vi "OP600ZP_GlobalVariables.vi"() -> ()   [LabVIEW 2020]
uses:
  CheminDeBase.vi
  <vilib>/Utility/config.llb/Read Key (Double).vi
  OP600ZP_VGConf.vi
  <vilib>/Utility/config.llb/Read Key (String).vi
  OP500/SubVI/OP500ZP_VGConf.vi
  <vilib>/Utility/config.llb/NI_LVConfig.lvlib
panel:
  out "error out 2":errorcluster caption="error out"
  out "error out":errorcluster
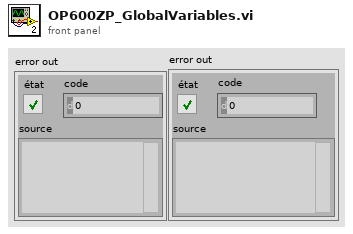
[diagram p1: front panel]
types:
  T1 = typedef "NI_LVConfig.lvlib/Config Data RefNum.ctl" = refnum<k1>
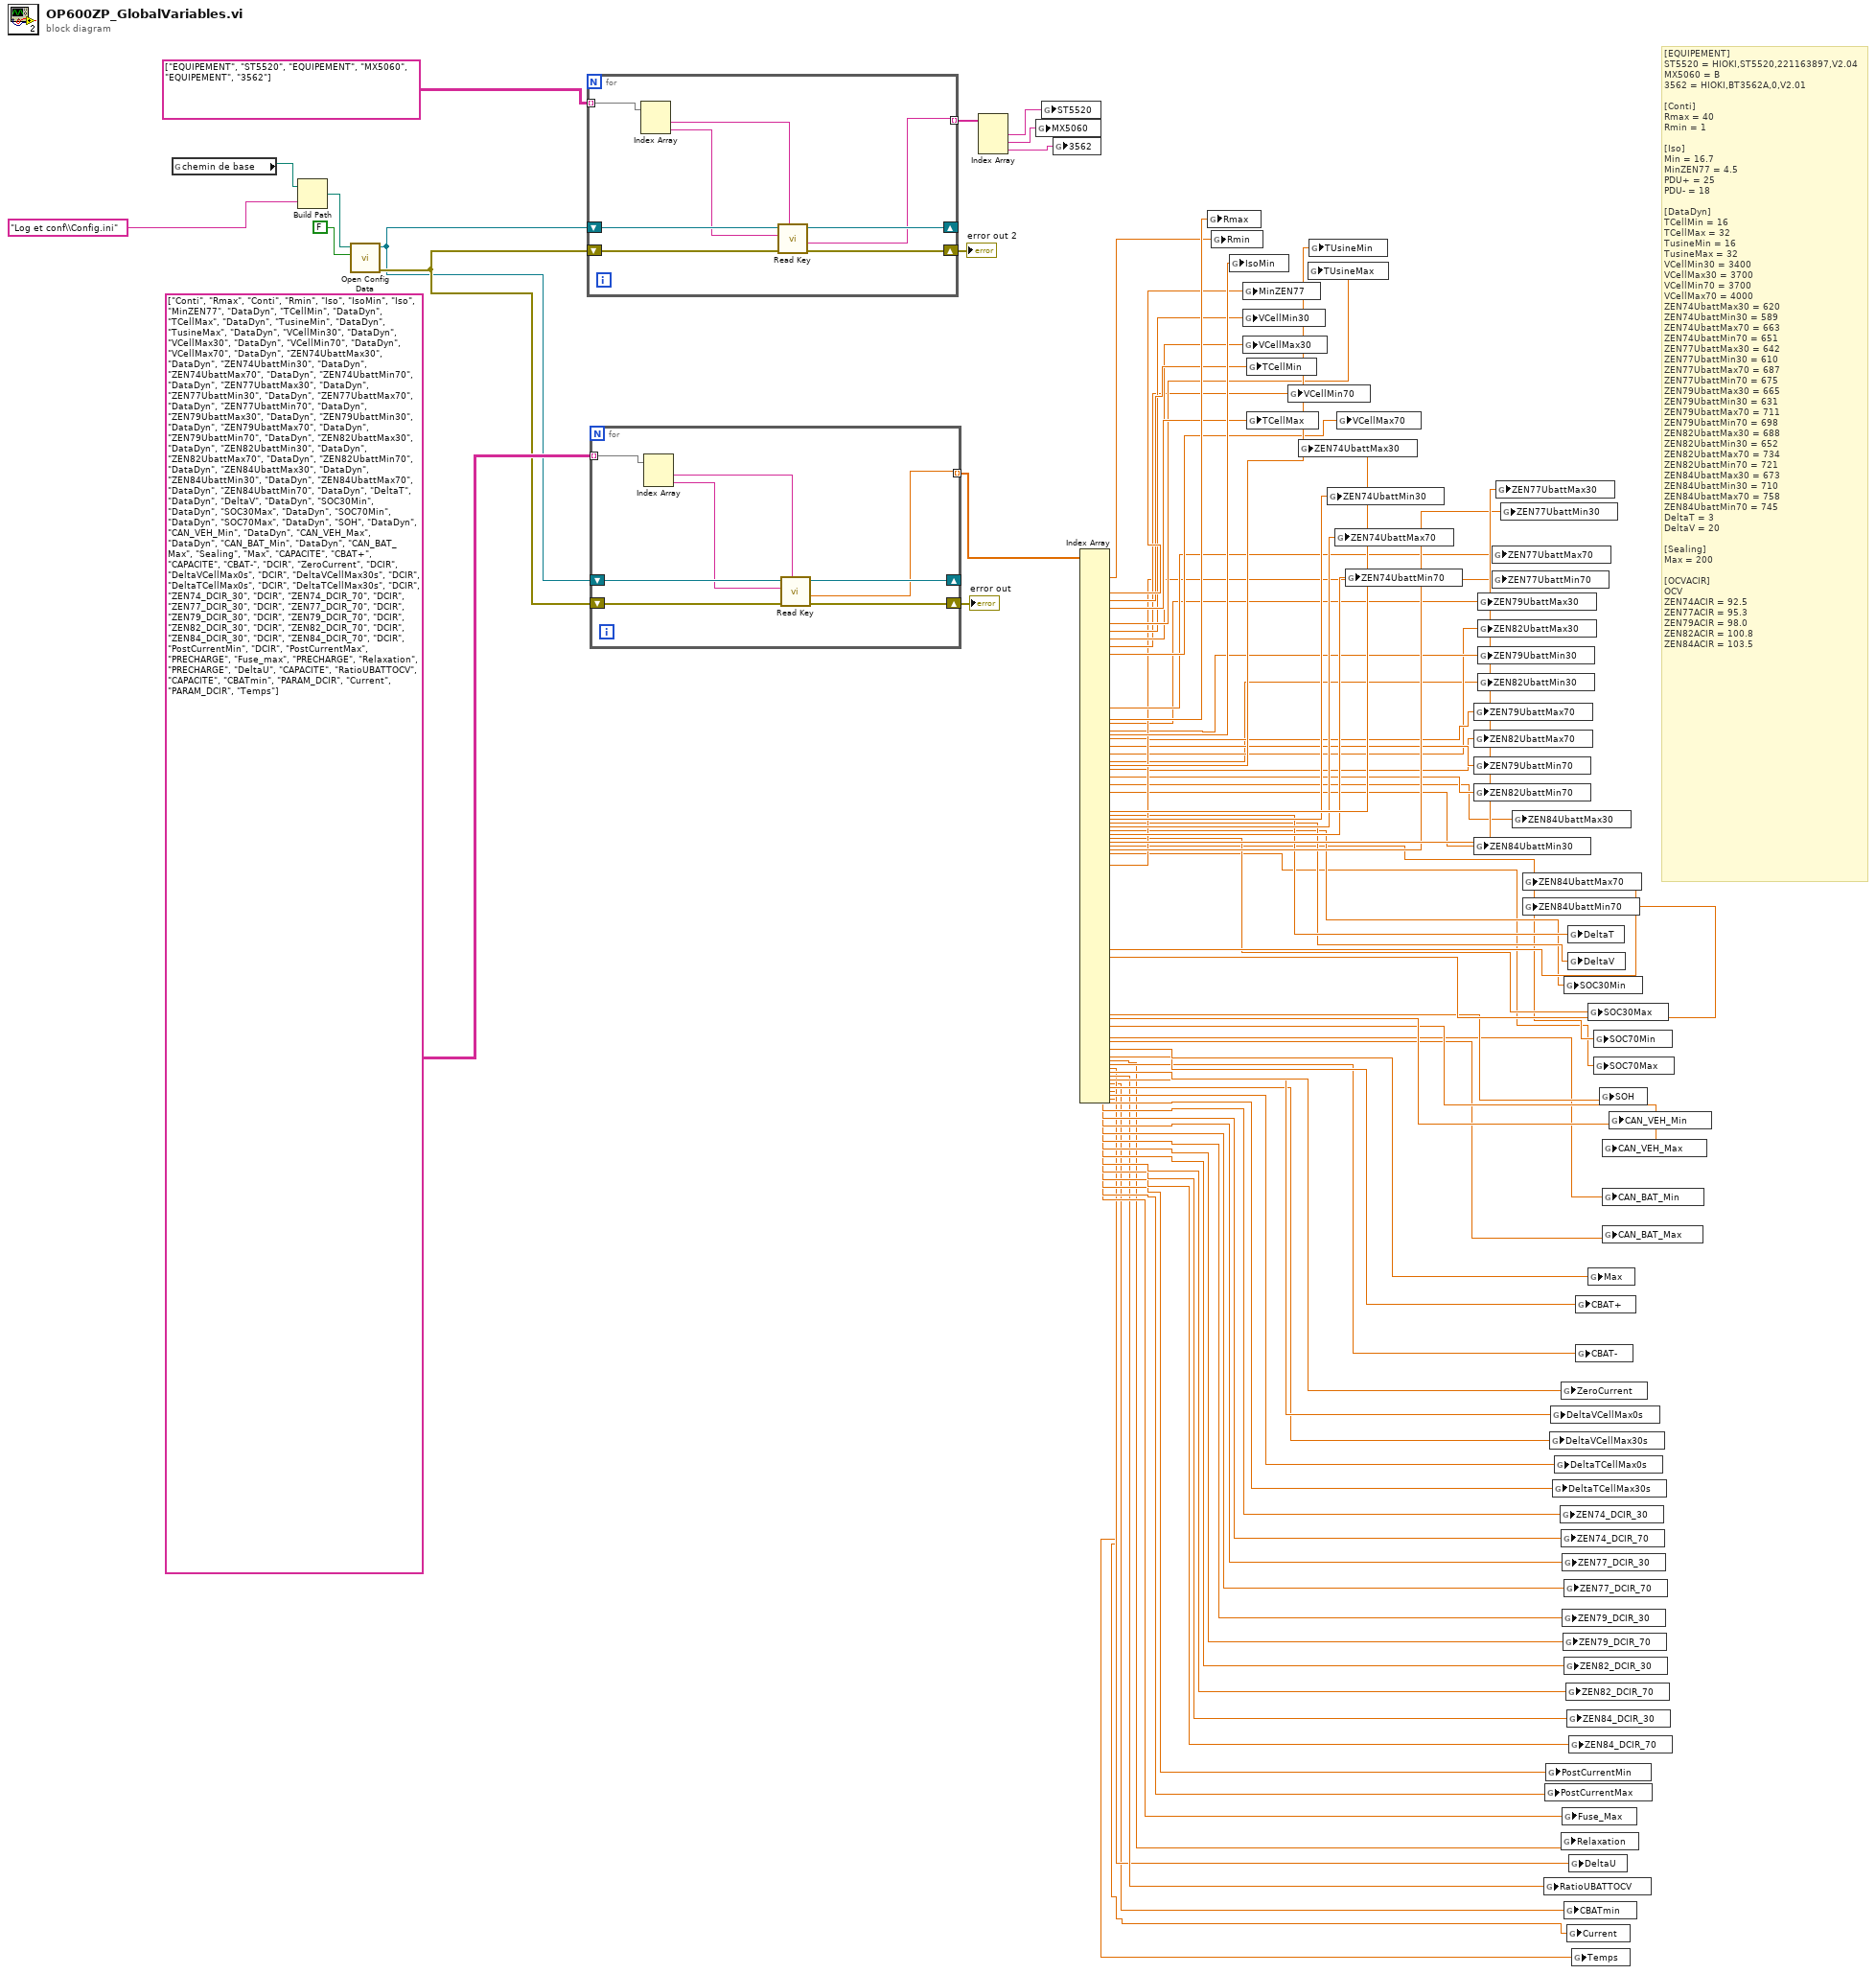
[diagram p0: block diagram]
diagram:
  # "[EQUIPEMENT]\nST5520 = HIOKI,ST5520,221163897,V2.04\t\nMX5060 = B\n3562 = HIOKI,BT3562A,0,V2.01\n\n[Conti]\nRmax = 40\nRmin = 1\n\n[Iso]\nMin = 16.7\nMinZEN77 = 4.5\nPDU+ = 25\nPDU- = 18\n\n[DataDyn]\nTCellMin = 16\nTCellMax = 32\nTusineMin = 16\nTusineMax = 32\nVCellMin30 = 3400\nVCellMax30 = 3700\nVCellMin70 = 3700\nVCellMax70 = 4000\nZEN74UbattMax30 = 620\nZEN74UbattMin30 = 589\nZEN74UbattMax70 = 663\nZEN74UbattMin70 = 651\nZEN77UbattMax30 = 642\nZEN77UbattMin30 = 610\nZEN77UbattMax70 = 687\nZEN77UbattMin70 = 675\nZEN79UbattMax30 = 665\nZEN79UbattMin30 = 631\nZEN79UbattMax70 = 711\nZEN79UbattMin70 = 698\nZEN82UbattMax30 = 688\nZEN82UbattMin30 = 652\nZEN82UbattMax70 = 734\nZEN82UbattMin70 = 721\nZEN84UbattMax30 = 673\nZEN84UbattMin30 = 710\nZEN84UbattMax70 = 758\nZEN84UbattMin70 = 745\nDeltaT = 3\nDeltaV = 20\n\n[Sealing]\nMax = 200\n\n[OCVACIR]\nOCV\nZEN74ACIR = 92.5\nZEN77ACIR = 95.3\nZEN79ACIR = 98.0\nZEN82ACIR = 100.8\nZEN84ACIR = 103.5"
  n1 = global read "CheminDeBase.vi" "chemin de base"() -> (w71:path)
  n2 = Build Path(base path=w71, name or relative path="Log et conf\\Config.ini") -> (appended path=w84:path)
  n3 = call <vilib>:"Open Config Data.vi"("create file if necessary (T)"=FALSE, "configuration file path"=w84) -> ("error out"=w75:errorcluster, "refnum"=w74:T1)  [unwired: 7 in, 1 out]
  n4 = for {
    tunnel: string[][] [["EQUIPEMENT", "ST5520"], ["EQUIPEMENT", "MX5060"], ["EQUIPEMENT", "3562"]] -> [w90] mode=indexing
    shift-right: [w91] -> w72
    shift-left: w75 -> [w93]
    shift-right: [w87] -> _
    shift-left: w74 -> [w92]
    tunnel: [w86] -> w81 mode=indexing
    n5 = Index Array(array=w90) -> (element #1=w89:string, element #2=w88:string)  [unwired: 2 in]
    n6 = call-poly <vilib>:"Read Key.vi"("section"=w89, "error in (no error)"=w93, "key"=w88, "refnum"=w92) -> ("error out"=w91:errorcluster, "value"=w86:string, "refnum out"=w87:T1)  [unwired: 4 in, 1 out]
  }
  "error out 2" <- w72
  n7 = for {
    tunnel: string[][] [["Conti", "Rmax"], ["Conti", "Rmin"], ["Iso", "IsoMin"], ["Iso", "MinZEN77"], ["DataDyn", "TCellMin"], ["DataDyn", "TCellMax"], ["DataDyn", "TusineMin"], ["DataDyn", "TusineMax"], ["DataDyn", "VCellMin30"], ["DataDyn", "VCellMax30"], ["DataDyn", "VCellMin70"], ["DataDyn", "VCellMax70"], ["DataDyn", "ZEN74UbattMax30"], ["DataDyn", "ZEN74UbattMin30"], ["DataDyn", "ZEN74UbattMax70"], ["DataDyn", "ZEN74UbattMin70"], ["DataDyn", "ZEN77UbattMax30"], ["DataDyn", "ZEN77UbattMin30"], ["DataDyn", "ZEN77UbattMax70"], ["DataDyn", "ZEN77UbattMin70"], ["DataDyn", "ZEN79UbattMax30"], ["DataDyn", "ZEN79UbattMin30"], ["DataDyn", "ZEN79UbattMax70"], ["DataDyn", "ZEN79UbattMin70"], ["DataDyn", "ZEN82UbattMax30"], ["DataDyn", "ZEN82UbattMin30"], ["DataDyn", "ZEN82UbattMax70"], ["DataDyn", "ZEN82UbattMin70"], ["DataDyn", "ZEN84UbattMax30"], ["DataDyn", "ZEN84UbattMin30"], ["DataDyn", "ZEN84UbattMax70"], ["DataDyn", "ZEN84UbattMin70"], ["DataDyn", "DeltaT"], ["DataDyn", "DeltaV"], ["DataDyn", "SOC30Min"], ["DataDyn", "SOC30Max"], ["DataDyn", "SOC70Min"], ["DataDyn", "SOC70Max"], ["DataDyn", "SOH"], ["DataDyn", "CAN_VEH_Min"], ["DataDyn", "CAN_VEH_Max"], ["DataDyn", "CAN_BAT_Min"], ["DataDyn", "CAN_BAT_Max"], ["Sealing", "Max"], ["CAPACITE", "CBAT+"], ["CAPACITE", "CBAT-"], ["DCIR", "ZeroCurrent"], ["DCIR", "DeltaVCellMax0s"], ["DCIR", "DeltaVCellMax30s"], ["DCIR", "DeltaTCellMax0s"], ["DCIR", "DeltaTCellMax30s"], ["DCIR", "ZEN74_DCIR_30"], ["DCIR", "ZEN74_DCIR_70"], ["DCIR", "ZEN77_DCIR_30"], ["DCIR", "ZEN77_DCIR_70"], ["DCIR", "ZEN79_DCIR_30"], ["DCIR", "ZEN79_DCIR_70"], ["DCIR", "ZEN82_DCIR_30"], ["DCIR", "ZEN82_DCIR_70"], ["DCIR", "ZEN84_DCIR_30"], ["DCIR", "ZEN84_DCIR_70"], ["DCIR", "PostCurrentMin"], ["DCIR", "PostCurrentMax"], ["PRECHARGE", "Fuse_max"], ["PRECHARGE", "Relaxation"], ["PRECHARGE", "DeltaU"], ["CAPACITE", "RatioUBATTOCV"], ["CAPACITE", "CBATmin"], ["PARAM_DCIR", "Current"], ["PARAM_DCIR", "Temps"]] -> [w98] mode=indexing
    shift-right: [w99] -> w73
    shift-left: w75 -> [w101]
    shift-right: [w95] -> _
    shift-left: w74 -> [w100]
    tunnel: [w94] -> w76 mode=indexing
    n8 = Index Array(array=w98) -> (element #1=w97:string, element #2=w96:string)  [unwired: 2 in]
    n9 = call-poly <vilib>:"Read Key.vi"("section"=w97, "error in (no error)"=w101, "key"=w96, "refnum"=w100) -> ("error out"=w99:errorcluster, "value"=w94:dbl, "refnum out"=w95:T1)  [unwired: 4 in, 1 out]
  }
  "error out" <- w73
  n10 = Index Array(array=w81) -> (element #1=w80:string, element #2=w79:string, element #3=w78:string)  [unwired: 3 in]
  n11 = global write "OP500ZP_VGConf.vi" "MX5060"(w79) -> ()
  n12 = global write "OP500ZP_VGConf.vi" "ST5520"(w80) -> ()
  n13 = global write "OP500ZP_VGConf.vi" "3562"(w78) -> ()
  n14 = Index Array(array=w76) -> (element #1=w70:dbl, element #2=w9:dbl, element #3=w69:dbl, element #4=w68:dbl, element #5=w67:dbl, element #6=w66:dbl, element #7=w65:dbl, element #8=w64:dbl, element #9=w63:dbl, element #10=w62:dbl, element #11=w61:dbl, element #12=w60:dbl, element #13=w59:dbl, element #14=w58:dbl, element #15=w57:dbl, element #16=w56:dbl, element #17=w55:dbl, element #18=w54:dbl, element #19=w53:dbl, element #20=w52:dbl, element #21=w51:dbl, element #22=w50:dbl, element #23=w49:dbl, element #24=w48:dbl, element #25=w47:dbl, element #26=w46:dbl, element #27=w45:dbl, element #28=w44:dbl, element #29=w43:dbl, element #30=w42:dbl, element #31=w41:dbl, element #32=w40:dbl, element #33=w39:dbl, element #34=w38:dbl, element #35=w37:dbl, element #36=w36:dbl, element #37=w35:dbl, element #38=w34:dbl, element #39=w33:dbl, element #40=w32:dbl, element #41=w31:dbl, element #42=w30:dbl, element #43=w29:dbl, element #44=w28:dbl, element #45=w27:dbl, element #46=w26:dbl, element #47=w25:dbl, element #48=w24:dbl, element #49=w23:dbl, element #50=w22:dbl, element #51=w21:dbl, element #52=w20:dbl, element #53=w19:dbl, element #54=w18:dbl, element #55=w17:dbl, element #56=w16:dbl, element #57=w15:dbl, element #58=w14:dbl, element #59=w13:dbl, element #60=w12:dbl, element #61=w11:dbl, element #62=w10:dbl, element #63=w8:dbl, element #64=w7:dbl, element #65=w6:dbl, element #66=w4:dbl, element #67=w5:dbl, element #68=w3:dbl, element #69=w2:dbl, element #70=w1:dbl)  [unwired: 70 in]
  n15 = global write "OP600ZP_VGConf.vi" "Rmax"(w70) -> ()
  n16 = global write "OP600ZP_VGConf.vi" "Rmin"(w9) -> ()
  n17 = global write "OP600ZP_VGConf.vi" "IsoMin"(w69) -> ()
  n18 = global write "OP600ZP_VGConf.vi" "MinZEN77"(w68) -> ()
  n19 = global write "OP600ZP_VGConf.vi" "VCellMin30"(w63) -> ()
  n20 = global write "OP600ZP_VGConf.vi" "VCellMax30"(w62) -> ()
  n21 = global write "OP600ZP_VGConf.vi" "TCellMin"(w67) -> ()
  n22 = global write "OP600ZP_VGConf.vi" "TCellMax"(w66) -> ()
  n23 = global write "OP600ZP_VGConf.vi" "VCellMin70"(w61) -> ()
  n24 = global write "OP600ZP_VGConf.vi" "ZEN74UbattMax30"(w59) -> ()
  n25 = global write "OP600ZP_VGConf.vi" "TUsineMax"(w64) -> ()
  n26 = global write "OP600ZP_VGConf.vi" "TUsineMin"(w65) -> ()
  n27 = global write "OP600ZP_VGConf.vi" "ZEN74UbattMin30"(w58) -> ()
  n28 = global write "OP600ZP_VGConf.vi" "ZEN74UbattMax70"(w57) -> ()
  n29 = global write "OP600ZP_VGConf.vi" "VCellMax70"(w60) -> ()
  n30 = global write "OP600ZP_VGConf.vi" "ZEN74UbattMin70"(w56) -> ()
  n31 = global write "OP600ZP_VGConf.vi" "ZEN79UbattMax70"(w49) -> ()
  n32 = global write "OP600ZP_VGConf.vi" "ZEN82UbattMax70"(w45) -> ()
  n33 = global write "OP600ZP_VGConf.vi" "ZEN79UbattMin70"(w48) -> ()
  n34 = global write "OP600ZP_VGConf.vi" "ZEN82UbattMin70"(w44) -> ()
  n35 = global write "OP600ZP_VGConf.vi" "ZEN84UbattMin30"(w42) -> ()
  n36 = global write "OP600ZP_VGConf.vi" "ZEN79UbattMax30"(w51) -> ()
  n37 = global write "OP600ZP_VGConf.vi" "ZEN82UbattMax30"(w47) -> ()
  n38 = global write "OP600ZP_VGConf.vi" "ZEN79UbattMin30"(w50) -> ()
  n39 = global write "OP600ZP_VGConf.vi" "ZEN82UbattMin30"(w46) -> ()
  n40 = global write "OP600ZP_VGConf.vi" "ZEN77UbattMax70"(w53) -> ()
  n41 = global write "OP600ZP_VGConf.vi" "ZEN77UbattMin70"(w52) -> ()
  n42 = global write "OP600ZP_VGConf.vi" "ZEN77UbattMax30"(w55) -> ()
  n43 = global write "OP600ZP_VGConf.vi" "ZEN77UbattMin30"(w54) -> ()
  n44 = global write "OP600ZP_VGConf.vi" "ZEN84UbattMax30"(w43) -> ()
  n45 = global write "OP600ZP_VGConf.vi" "ZEN84UbattMax70"(w41) -> ()
  n46 = global write "OP600ZP_VGConf.vi" "ZEN84UbattMin70"(w40) -> ()
  n47 = global write "OP600ZP_VGConf.vi" "RatioUBATTOCV"(w5) -> ()
  n48 = global write "OP600ZP_VGConf.vi" "PostCurrentMax"(w8) -> ()
  n49 = global write "OP600ZP_VGConf.vi" "PostCurrentMin"(w10) -> ()
  n50 = global write "OP600ZP_VGConf.vi" "DeltaVCellMax30s"(w23) -> ()
  n51 = global write "OP600ZP_VGConf.vi" "DeltaVCellMax0s"(w24) -> ()
  n52 = global write "OP600ZP_VGConf.vi" "DeltaTCellMax30s"(w21) -> ()
  n53 = global write "OP600ZP_VGConf.vi" "DeltaTCellMax0s"(w22) -> ()
  n54 = global write "OP600ZP_VGConf.vi" "ZEN74_DCIR_30"(w20) -> ()
  n55 = global write "OP600ZP_VGConf.vi" "ZeroCurrent"(w25) -> ()
  n56 = global write "OP600ZP_VGConf.vi" "ZEN74_DCIR_70"(w19) -> ()
  n57 = global write "OP600ZP_VGConf.vi" "Relaxation"(w6) -> ()
  n58 = global write "OP600ZP_VGConf.vi" "ZEN77_DCIR_30"(w18) -> ()
  n59 = global write "OP600ZP_VGConf.vi" "ZEN79_DCIR_30"(w16) -> ()
  n60 = global write "OP600ZP_VGConf.vi" "Fuse_Max"(w7) -> ()
  n61 = global write "OP600ZP_VGConf.vi" "ZEN79_DCIR_70"(w15) -> ()
  n62 = global write "OP600ZP_VGConf.vi" "SOC30Min"(w37) -> ()
  n63 = global write "OP600ZP_VGConf.vi" "ZEN77_DCIR_70"(w17) -> ()
  n64 = global write "OP600ZP_VGConf.vi" "ZEN82_DCIR_30"(w14) -> ()
  n65 = global write "OP600ZP_VGConf.vi" "CBATmin"(w3) -> ()
  n66 = global write "OP600ZP_VGConf.vi" "ZEN82_DCIR_70"(w13) -> ()
  n67 = global write "OP600ZP_VGConf.vi" "ZEN84_DCIR_30"(w12) -> ()
  n68 = global write "OP600ZP_VGConf.vi" "Current"(w2) -> ()
  n69 = global write "OP600ZP_VGConf.vi" "DeltaT"(w39) -> ()
  n70 = global write "OP600ZP_VGConf.vi" "DeltaV"(w38) -> ()
  n71 = global write "OP600ZP_VGConf.vi" "ZEN84_DCIR_70"(w11) -> ()
  n72 = global write "OP600ZP_VGConf.vi" "DeltaU"(w4) -> ()
  n73 = global write "OP600ZP_VGConf.vi" "Temps"(w1) -> ()
  n74 = global write "OP600ZP_VGConf.vi" "CBAT+"(w27) -> ()
  n75 = global write "OP600ZP_VGConf.vi" "CBAT-"(w26) -> ()
  n76 = global write "OP600ZP_VGConf.vi" "SOC30Max"(w36) -> ()
  n77 = global write "OP600ZP_VGConf.vi" "Max"(w28) -> ()
  n78 = global write "OP600ZP_VGConf.vi" "SOC70Min"(w35) -> ()
  n79 = global write "OP600ZP_VGConf.vi" "SOC70Max"(w34) -> ()
  n80 = global write "OP600ZP_VGConf.vi" "SOH"(w33) -> ()
  n81 = global write "OP600ZP_VGConf.vi" "CAN_VEH_Max"(w31) -> ()
  n82 = global write "OP600ZP_VGConf.vi" "CAN_BAT_Min"(w30) -> ()
  n83 = global write "OP600ZP_VGConf.vi" "CAN_BAT_Max"(w29) -> ()
  n84 = global write "OP600ZP_VGConf.vi" "CAN_VEH_Min"(w32) -> ()
